vi "generate engine info struct.vi"(8 "error in (no error)":errorcluster, 11 "shared memory editor node in":refnum<class "module editor node.lvclass">) -> (0 "error out":errorcluster, 2 "struct string":string, 3 "shared memory editor node out":refnum<class "module editor node.lvclass">)   [LabVIEW 2013, in "Shared Memory editor node.lvclass"]
uses:
  Shared Memory editor node.lvclass
  <vilib>/NI/DCAF/Tag Editor Core/Configuration Editor/Classes/Module editor node/module editor node.lvclass
  cheddar/C Header Generator.lvlib
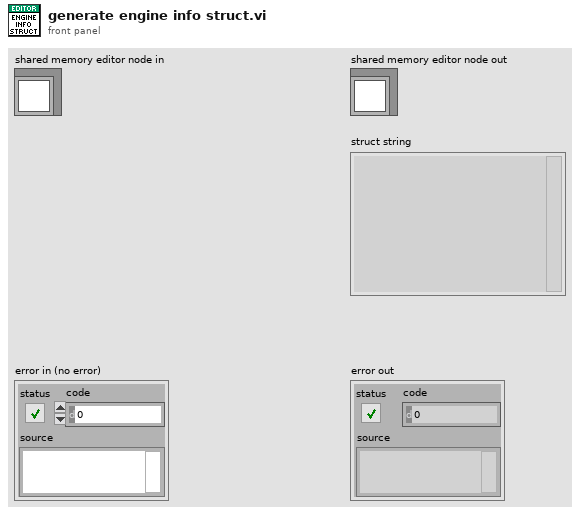
[diagram p1: front panel]
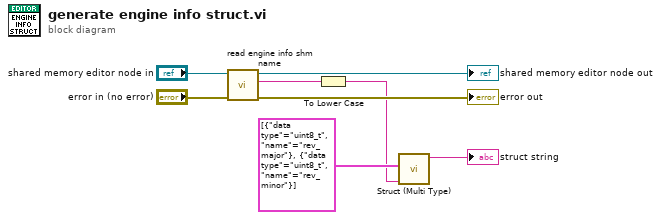
[diagram p0: block diagram]
diagram:
  n1 = call "read engine info shm name.vi"("error in"="error in (no error)", "shared memory editor node"="shared memory editor node in") -> ("error out"=→"error out":errorcluster, "shm name"=w1:string, "shared memory editor node out"=→"shared memory editor node out":refnum<class "module editor node.lvclass">)  [unwired: 7 in]
  n2 = To Lower Case(string=w1) -> (all lower case string=w2:string)
  n3 = call "Struct (Multi Type).vi"("Struct name"=w2, "Variables"=cluster{"data type":string, "name":string}[] [{"data type"="uint8_t", "name"="rev_major"}, {"data type"="uint8_t", "name"="rev_minor"}]) -> ("String out"=→"struct string":string)  [unwired: 9 in]
